vi "MVP02.vi"() -> ()   [LabVIEW 2016]
uses:
  Controls/Teste Case Selector 01.ctl
  <vilib>/xnet/xnet.llb/XNET Create Session (Frame Input Single-point).vi
  <vilib>/xnet/xnet.llb/XNET Write (Signal Single-point).vi
  <vilib>/xnet/xnet.llb/XNET Read (Signal Single-point).vi
panel:
  out "Waveform Chart":dbl(graph)
  out "String":string
  out "String (OCR/OCV 1)":string
  out "Passed?":bool
  in  "Menu":dbl[](array[numeric])=[0.0]
  in  "milliseconds to wait":u32=100
  in  "stop":bool
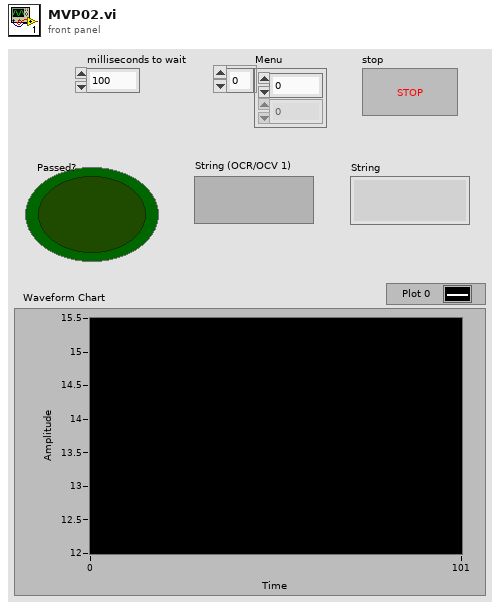
[diagram p1: front panel]
types:
  T1 = typedef "Teste Case Selector 01.ctl" = enum16{"Outros", "Caso 2,Valor 1", "Caso 2,Valor 2"}
  T2 = typedef "IMAQ Image.ctl" = refnum<image>
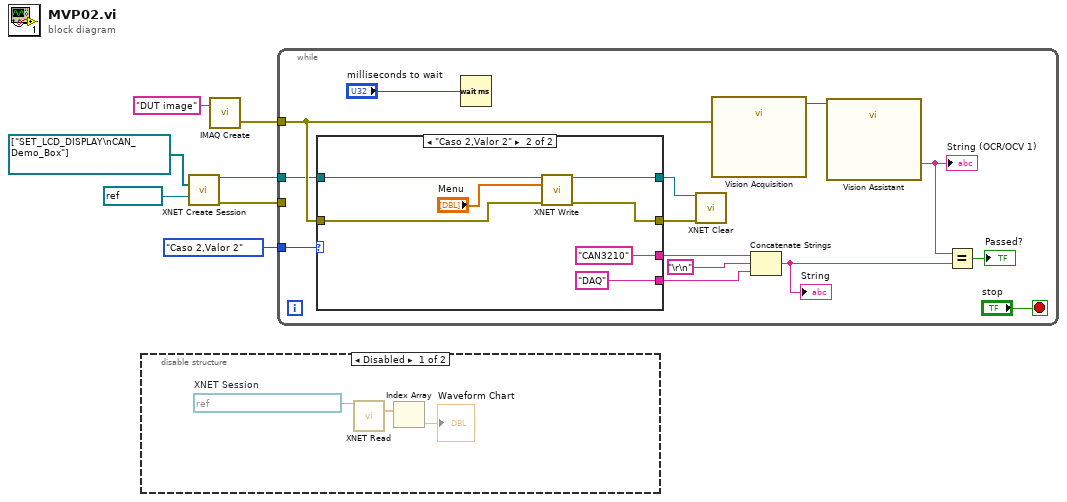
[diagram p0: block diagram]
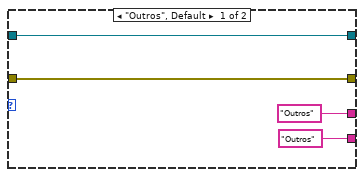
[diagram p3: hidden frame]
diagram:
  n1 = disable-structure shown="Disabled" {
    frame Disabled {
      w8 = refnum<k21> "Analog In To CAN Ch1"  # XNET Session
      n2 = call-poly <vilib>:"XNET Read.vi"("session in"=w8) -> ("data"=w9:dbl[])  [unwired: 12 in, 2 out]
      n3 = Index Array(array=w9) -> (element=→"Waveform Chart":dbl)  [unwired: 1 in]
    }
    frame Enabled {
    }
  }
  n4 = call-poly <vilib>:"XNET Create Session.vi"("frame list"=refnum<k21>[] ["SET_LCD_DISPLAY\nCAN_Demo_Box"], "interface"=refnum<k21> "CAN1") -> ("session out"=w3:refnum<k21>, "error out"=w2:errorcluster)  [unwired: 12 in]
  n5 = call "IMAQ Create"("Image Name"="DUT image") -> ("error out"=w5:errorcluster)  [unwired: 4 in, 1 out]
  n6 = while {
    tunnel: Teste_Case_Selector_01."Caso 2,Valor 2" -> [w22]
    tunnel: w5 -> [w12]
    tunnel: w3 -> [w11]
    tunnel: w2 -> [_]
    stop <- "stop" stop-if-true
    n7 = case shown="\"Caso 2,Valor 2\"" w22 {
      tunnel: ["Outros" "CAN3210"] -> w17
      tunnel: ["Outros" "DAQ"] -> w15
      tunnel: [w26 w32] -> w14
      tunnel: [w25 w31] -> w13
      tunnel: w12 -> [w26 w30]
      tunnel: w11 -> [w25 w29]
      frame "Outros", Default {
      }
      frame "Caso 2,Valor 2" {
        n8 = call-poly <vilib>:"XNET Write.vi"("session in"=w29, "data"="Menu", "error in (no error)"=w30) -> ("session out"=w31:refnum<k21>, "error out"=w32:errorcluster)  [unwired: 11 in]
      }
    }
    n9 = Wait (ms)(milliseconds to wait="milliseconds to wait") -> ()  [unwired: 1 out]
    n10 = call <vilib>:"XNET Clear.vi"("session in"=w13, "error in (no error)"=w14) -> ()  [unwired: 13 in, 1 out]
    n11 = call "Vision Acquisition"("error in"=w12) -> ("Image Out"=w19:T2)  [unwired: 25 in, 1 out]
    n12 = Concatenate Strings(w17, "\r\n", w15) -> (w18:string)
    "String" <- w18
    n13 = call "Vision Assistant"("Image In"=w19) -> ("String (OCR/OCV 1)"=w21:string)  [unwired: 24 in, 2 out]
    "String (OCR/OCV 1)" <- w21
    n14 = Equal?(x=w21, y=w18) -> (x = y?=→"Passed?":bool)
  }
